vi "Receive Update from Motors.vi"(8 "error in (no error)":errorcluster, 10 "Motors with Encoder State":T1={"Forward Switch"=FALSE, "Reverse Switch"=FALSE, "Measured RPM"=0.0, "Distance (in)"=0.0, "Setpoint RPM"=0.0, "Encoder Count"=0, "Home Count"=0, "Config"={"Counts  Per Revolution"=0, "Invert Encoder Direction"=FALSE, "Diameter of Revolution"=0.0, "Max RPM"=0.0, "Encoder Control"=TRUE}}, 11 "Receive Updates from Motors with Encoders in":refnum<class "Receive Updates from Motors with Encoders.lvclass">) -> (0 "error out":errorcluster, 3 "Receive Updates from Motors with Encoders out":refnum<class "Receive Updates from Motors with Encoders.lvclass">)   [LabVIEW 2014, in "Comp Motors with Encoders.lvlib" / "Receive Updates from Motors with Encoders.lvclass"]
uses:
  Receive Updates from Motors with Encoders.lvclass
  Robot/Motor with Encoders/Motors with Encoders Class/Motors with Encoders State.ctl
  Robot/Motor with Encoders/Motors with Encoders Class/Motors with Encoders Config.ctl
  Receive Updates from Motors with Encoders.lvclass/Receive Updates from Motors with Encoders.ctl
  Robot/Motor with Encoders/Motors with Encoders Class/Motors with Encoders.lvclass
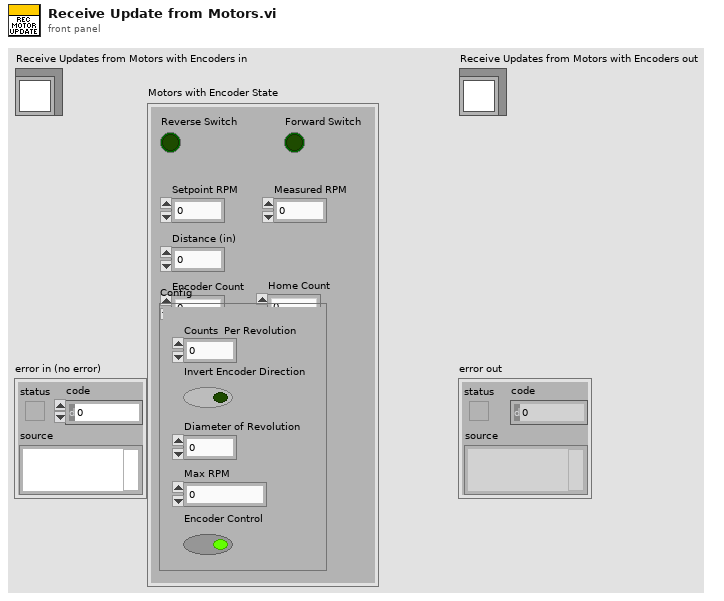
[diagram p1: front panel]
types:
  T1 = typedef "Motors with Encoders.lvlib/Motors with Encoders.lvclass/Motors with Encoders State.ctl" = cluster{"Forward Switch":bool, "Reverse Switch":bool, "Measured RPM":dbl, "Distance (in)":dbl, "Setpoint RPM":dbl, "Encoder Count":i64, "Home Count":i64, "Config":T2}
  T2 = typedef "Motors with Encoders.lvlib/Motors with Encoders.lvclass/Motors with Encoders Config.ctl" = cluster{"Counts  Per Revolution":u32, "Invert Encoder Direction":bool, "Diameter of Revolution":dbl, "Max RPM":dbl, "Encoder Control":bool}
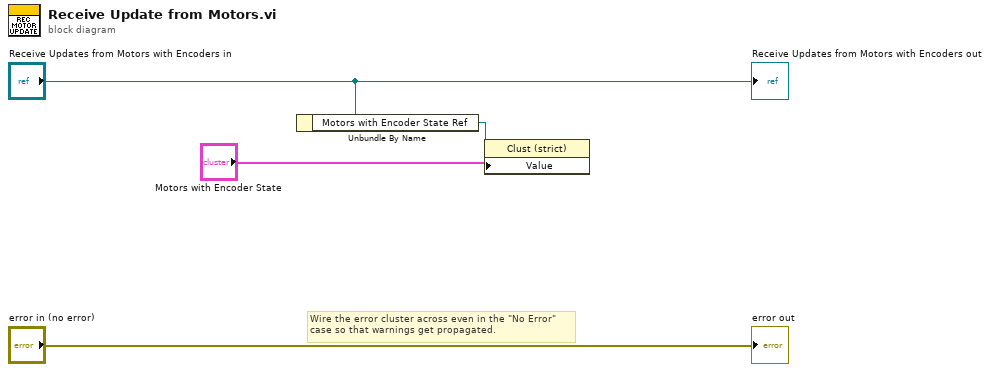
[diagram p0: block diagram]
diagram:
  # "Wire the error cluster across even in the \"No Error\"\ncase so that warnings get propagated."
  n1 = Unbundle By Name("Receive Updates from Motors with Encoders in") -> ("Motors with Encoder State Ref"=w2:refnum<vi>)
  n2 = property class="Clust (strict)"(reference=w2, "Value"="Motors with Encoder State") -> ()  [unwired: 1 in, 2 out]
  "error out" <- "error in (no error)"
  "Receive Updates from Motors with Encoders out" <- "Receive Updates from Motors with Encoders in"
